vi "Confirm USB Devices and IO.vi"() -> (1 "Device Name":string[](array[string])=["", "", "", "", "\n"], 2 "Num Dev":u32, 3 "Device Address":refnum<visa-resource-name>[](array[refnum]))   [LabVIEW 2024]
uses:
  <vilib>/Instr/_visa.llb/VISA Configure Serial Port (Instr).vi
panel:
  out "Communication Status":string[](array[string])=["", "", "", "", "\n"]
  out "Detection Status":string="1 devices detected"
  in  "stop":bool
  out "Detected USB Device Address":string[](array[string])=["ASRL10::INSTR"]
  # "USB Device Detection Service"
  # "If a device is not detected, unplug the missing device and replug it..."
  # "Ensure the models you want to use are present in the list"
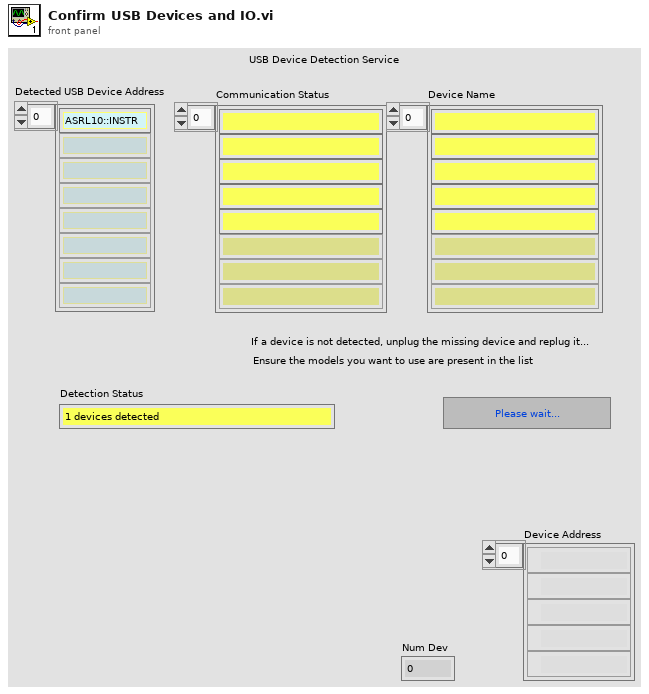
[diagram p1: front panel]
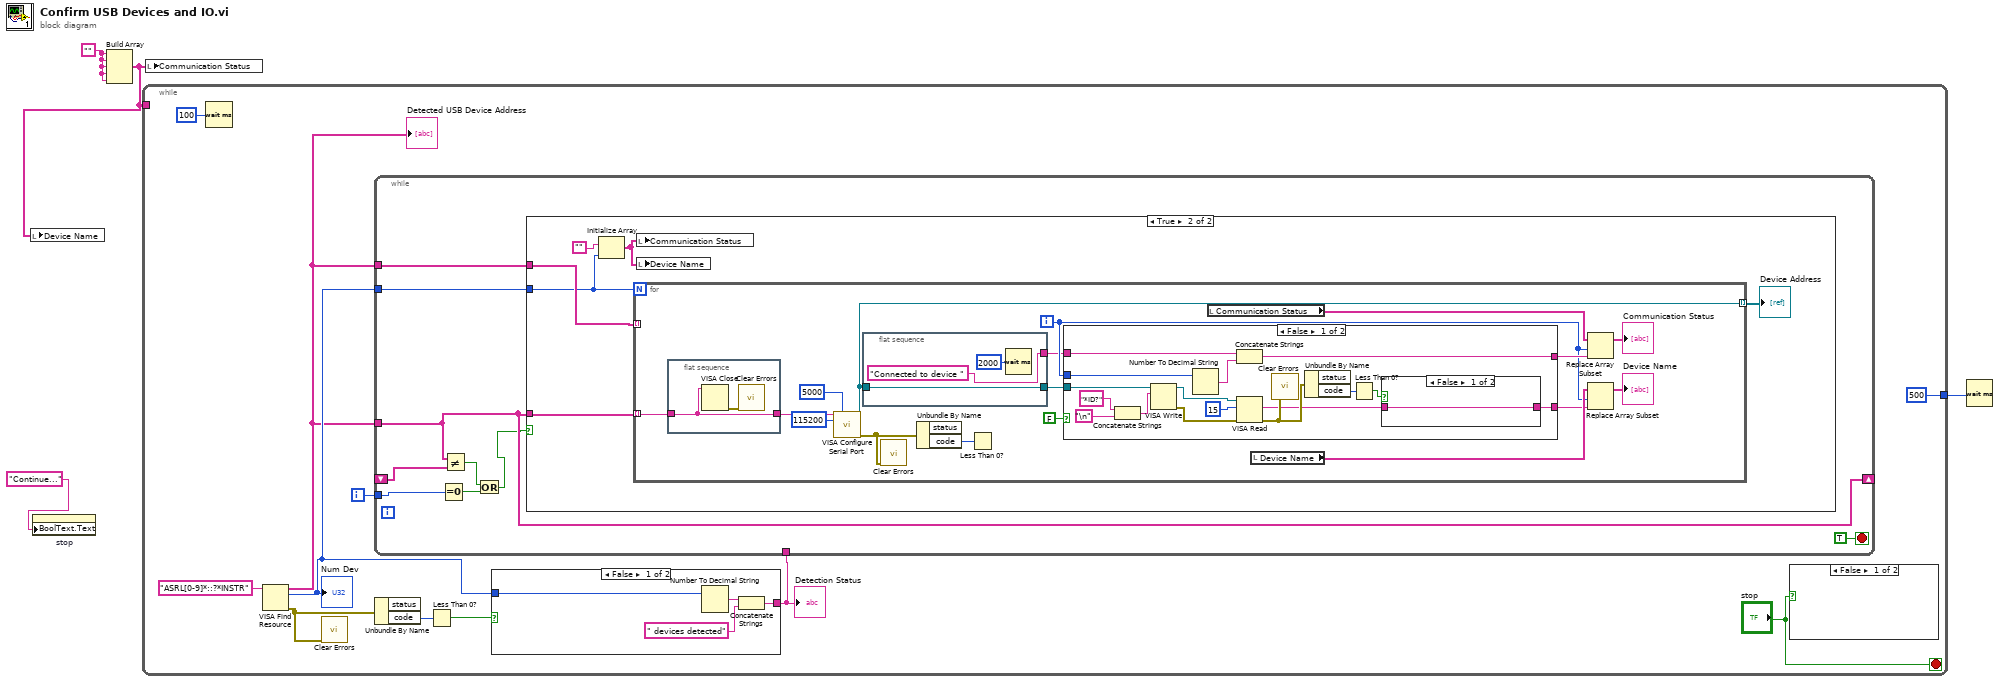
[diagram p0: block diagram]
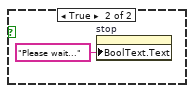
[diagram p2: hidden frame]
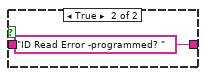
[diagram p4: hidden frame]
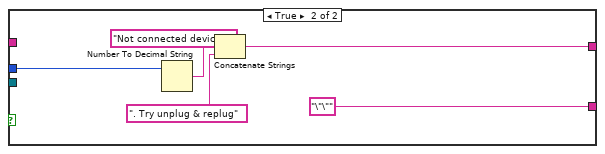
[diagram p5: hidden frame]
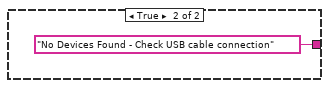
[diagram p6: hidden frame]
diagram:
  w4 = ""
  n1 = property on="stop" class="Bool"("BoolText.Text"="Continue..." ("Boolean Text.Text")) -> ()  [unwired: 2 in, 2 out]
  n2 = Build Array(w4, w4, w4, w4, w4) -> (w1:string[])
  n3 = local write "Device Name"(w1) -> ()
  n4 = while {
    tunnel: w1 -> [_]
    tunnel: [u32 500 ("milliseconds to wait")] -> w3
    i -> [w7]
    stop <- "stop" stop-if-true
    n5 = Wait (ms)(milliseconds to wait=u32 100) -> ()  [unwired: 1 out]
    n6 = VISA Find Resource(11:"ASRL[0-9]*::?*INSTR" ("expression (\"?*\")")) -> (0:w9:errorcluster, 2:w6:u32, 3:w5:string[])  [unwired: 2 in]
    "Detected USB Device Address" <- w5
    "Num Dev" <- w6
    n7 = call <vilib>:"Clear Errors.vi"("error in (no error)"=w9) -> ()  [unwired: 5 in, 2 out]
    n8 = Unbundle By Name(w9) -> ("code"=w14:i32)  [unwired: 1 out]
    n9 = Less Than 0?(x=w14) -> (x < 0?=w13:bool)
    n10 = case shown="False" w13 {
      tunnel: [w78 "No Devices Found - Check USB cable connection"] -> w8
      tunnel: w6 -> [w81 _]
      frame False {
        n11 = Number To Decimal String(number=w81) -> (decimal integer string=w80:string)  [unwired: 1 in]
        n12 = Concatenate Strings(w80, " devices detected") -> (w78:string)
      }
      frame True {
      }
    }
    "Detection Status" <- w8
    n13 = while {
      shift-right: [w24] -> _
      shift-left: _ -> [w23]
      tunnel: w5 -> [w24]
      tunnel: w7 -> [w22]
      tunnel: w8 -> [_]
      tunnel: w6 -> [w18]
      tunnel: w5 -> [w17]
      stop <- TRUE stop-if-true
      n14 = Equal To 0?(x=w22) -> (x = 0?=w21:bool)
      n15 = Not Equal?(x=w24, y=w23) -> (x != y?=w20:bool)
      n16 = Or(x=w20, y=w21) -> (x .or. y?=w19:bool)
      n17 = case shown="True" w19 {
        tunnel: w24 -> [_ w31]
        tunnel: w18 -> [_ w26]
        tunnel: w17 -> [_ w29]
        frame False {
        }
        frame True {
          n18 = Initialize Array("", w26) -> (w27:string[])
          n19 = for {
            N: w26 -> [_]
            tunnel: w31 -> [w46] mode=indexing
            tunnel: [w35] -> w30 mode=indexing
            tunnel: w29 -> [_] mode=indexing
            i -> [w40]
            n20 = flat-sequence {
              tunnel: w46 -> [w53]
              tunnel: [w53] -> w45
              frame #0 {
                n21 = VISA Close(VISA resource name=w53) -> (error out=w52:errorcluster)  [unwired: 1 in]
                n22 = call <vilib>:"Clear Errors.vi"("error in (no error)"=w52) -> ()  [unwired: 5 in, 2 out]
              }
            }
            n23 = call-poly "VISA Configure Serial Port"("VISA resource name"=w45, "timeout (10sec)"=u32 5000, "baud rate (9600)"=u32 115200) -> ("VISA resource name out"=w35:refnum<visa-resource-name>, "error out"=w47:errorcluster)  [unwired: 11 in]
            n24 = flat-sequence {
              tunnel: w35 -> [w50]
              tunnel: [w50] -> w36
              tunnel: ["Connected to device "] -> w32
              frame #0 {
                n25 = Wait (ms)(milliseconds to wait=u32 2000) -> ()  [unwired: 1 out]
              }
            }
            n26 = call <vilib>:"Clear Errors.vi"("error in (no error)"=w47) -> ()  [unwired: 5 in, 2 out]
            n27 = Unbundle By Name(w47) -> ("code"=w48:i32)  [unwired: 1 out]
            n28 = Less Than 0?(x=w48) -> ()  [unwired: 1 out]
            n29 = case shown="False" FALSE {
              tunnel: w40 -> [w68 w74]
              tunnel: [w67 w73] -> w43
              tunnel: [w56 "\"\"" ("read buffer")] -> w39
              tunnel: w36 -> [w60 _]
              tunnel: w32 -> [w54 _]
              frame False {
                n30 = Concatenate Strings("*ID?", "\n") -> (w61:string)
                n31 = VISA Write(VISA resource name=w60, write buffer=w61) -> (VISA resource name out=w65:refnum<visa-resource-name>, error out=w66:errorcluster)  [unwired: 1 in, 1 out]
                n32 = Number To Decimal String(number=w68) -> (decimal integer string=w69:string)  [unwired: 1 in]
                n33 = Concatenate Strings(w54, w69) -> (w67:string)
                n34 = VISA Read(VISA resource name=w65, byte count=u32 15, error in (no error)=w66) -> (read buffer=w57:string, error out=w58:errorcluster)  [unwired: 2 out]
                n35 = call <vilib>:"Clear Errors.vi"("error in (no error)"=w58) -> ()  [unwired: 5 in, 2 out]
                n36 = Unbundle By Name(w58) -> ("code"=w59:i32)  [unwired: 1 out]
                n37 = Less Than 0?(x=w59) -> (x < 0?=w55:bool)
                n38 = case shown="False" w55 {
                  tunnel: [w70 "ID Read Error -programmed? " ("read buffer")] -> w56
                  tunnel: w57 -> [w70 _]
                  frame False {
                  }
                  frame True {
                  }
                }
              }
              frame True {
                n39 = Number To Decimal String(number=w74) -> (decimal integer string=w76:string)  [unwired: 1 in]
                n40 = Concatenate Strings("Not connected device ", w76, ". Try unplug & replug") -> (w73:string)
              }
            }
            n41 = local read "Communication Status"() -> (w44:string[])
            n42 = local read "Device Name"() -> (w41:string[])
            n43 = Replace Array Subset(array=w44, new element=w43, index=w40) -> (→"Communication Status":string[])
            n44 = Replace Array Subset(array=w41, new element=w39, index=w40) -> (→"Device Name":string[])
          }
          "Device Address" <- w30
          n45 = local write "Communication Status"(w27) -> ()
          n46 = local write "Device Name"(w27) -> ()
        }
      }
    }
    n47 = case shown="False" "stop" {
      frame False {
      }
      frame True {
        n48 = property on="stop" class="Bool"("BoolText.Text"="Please wait..." ("Label.Text")) -> ()  [unwired: 2 in, 2 out]
      }
    }
  }
  n49 = local write "Communication Status"(w1) -> ()
  n50 = Wait (ms)(milliseconds to wait=w3) -> ()  [unwired: 1 out]
